vi "Example_IV_Curves.vi"() -> ()   [LabVIEW 2016]
uses:
  LockinDAQ/Typedefs/AO-cluster.ctl
  LockinDAQ/Typedefs/Function-enum.ctl
  Instrument.Lockin/Instrument.Lockin.lvclass
  <userlib>/LevyLab/LV to ITX/LVtoITX.lvclass
  LockinDAQ/Typedefs/AO_Channel-Numeric.ctl
  LockinDAQ/LockinDAQ.lvclass
panel:
  out "2 terminal":cluster{"Y":dbl[], "Y":dbl[]}(graph)
  out "4 terminal":cluster{"Y":dbl[], "Y":dbl[]}(graph)
  in  "step":dbl=0.025
  in  "end":dbl=0.1
  in  "start":dbl
  in  "Channels: AO":T1 {"f (Hz)" min=0.001 max=10000.0 format="%.3g"; "Phase (°)" format="%.3g"; "DC (V)" format="%.3p"; "Amp (V)" min=0.0 max=10.0 format="%.3p"}
  # "Lockin Example: IV Curves\nMake Sure Lockin Program is running!"
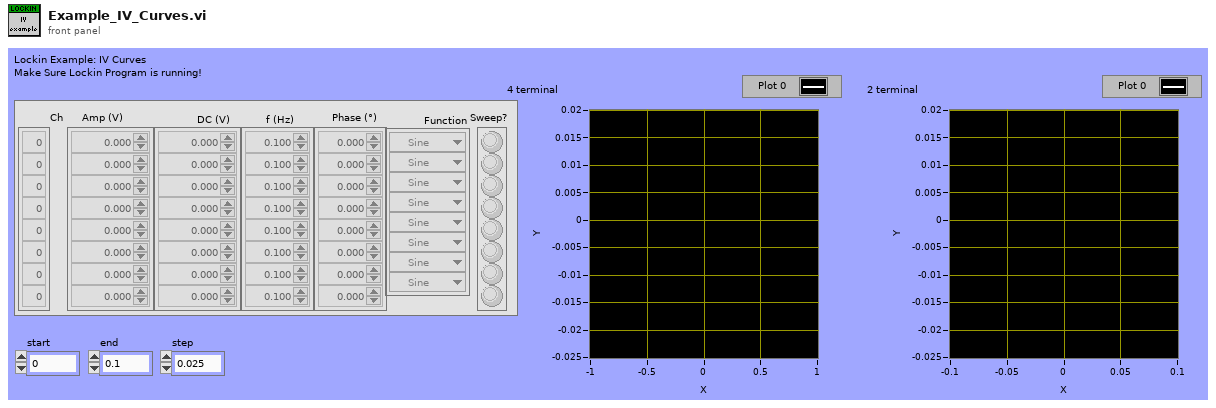
[diagram p1: front panel]
types:
  T1 = typedef "LockinDAQ.lvclass/AO-cluster.ctl" = cluster{"Ch":i32[], "Amp (V)":dbl[], "DC (V)":dbl[], "f (Hz)":dbl[], "Phase (°)":dbl[], "Function":T2[], "Sweep?":bool[]}
  T2 = typedef "LockinDAQ.lvclass/Function-enum.ctl" = enum16{"Sine", "Triangle", "Square", "Sawtooth"}
  T3 = typedef "LockinDAQ.lvclass/AO_Channel-Numeric.ctl" = i32
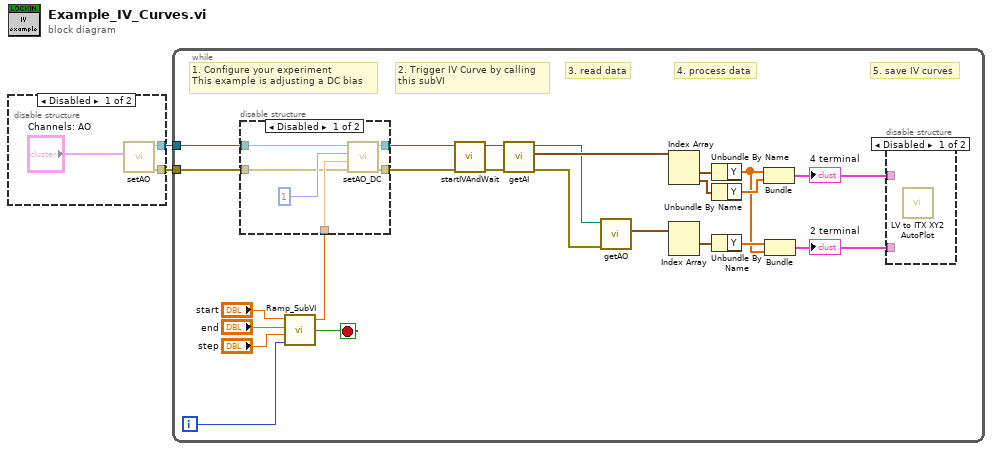
[diagram p0: block diagram]
diagram:
  n1 = disable-structure shown="Disabled" {
    disable-tunnel: [w4 _] -> w2
    disable-tunnel: [w3 _] -> w1
    frame Disabled {
      n2 = call "setAO.vi"("Channels: AO"="Channels: AO") -> ("error out"=w3:errorcluster, "Instrument.Lockin out"=w4:refnum<class "Instrument.Lockin.lvclass">)  [unwired: 9 in]
    }
    frame Enabled {
    }
  }
  n3 = while {
    tunnel: w2 -> [w14]
    tunnel: w1 -> [w13]
    i -> [w26]
    stop <- w29 stop-if-true
    # "5. save IV curves"
    # "4. process data"
    # "3. read data"
    # "1. Configure your experiment\nThis example is adjusting a DC bias"
    # "2. Trigger IV Curve by calling\nthis subVI"
    n4 = call <userlib>:"Ramp_SubVI.vi"("index"=w26, "step"="step", "end"="end", "start"="start") -> ("Stop?"=w29:bool, "Numeric"=w17:dbl)  [unwired: 1 in]
    n5 = disable-structure shown="Disabled" {
      disable-tunnel: w17 -> [w35 _]
      disable-tunnel: w14 -> [w33 _]
      disable-tunnel: w13 -> [w32 _]
      disable-tunnel: [w31 _] -> w12
      disable-tunnel: [w30 _] -> w11
      frame Disabled {
        n6 = call "setAO_DC.vi"("error in (no error)"=w32, "DC (V)"=w35, "AO Channel"=T3 1, "Instrument.Lockin in"=w33) -> ("error out"=w31:errorcluster, "Instrument.Lockin out"=w30:refnum<class "Instrument.Lockin.lvclass">)  [unwired: 6 in]
      }
      frame Enabled {
      }
    }
    n7 = call "startIVAndWait.vi"("error in (no error)"=w12, "Instrument.Lockin in"=w11) -> ("error out"=w9:errorcluster, "Instrument.Lockin out"=w10:refnum<class "Instrument.Lockin.lvclass">)  [unwired: 7 in, 1 out]
    n8 = call "getAI.vi"("error in (no error)"=w9, "Instrument.Lockin in"=w10) -> ("error out"=w8:errorcluster, "AI Waveform"=w15:waveform(dbl)[], "Instrument.Lockin out"=w7:refnum<class "Instrument.Lockin.lvclass">)  [unwired: 7 in]
    n9 = call "getAO.vi"("error in (no error)"=w8, "Instrument.Lockin in"=w7) -> ("AO Waveforrm"=w16:waveform(dbl)[])  [unwired: 7 in, 2 out]
    n10 = Index Array(array=w15) -> (element #1=w24:waveform(dbl), element #2=w23:waveform(dbl))  [unwired: 2 in]
    n11 = Index Array(array=w16) -> (element #1=w22:waveform(dbl))  [unwired: 2 in, 1 out]
    n12 = Unbundle By Name(w24) -> ("Y"=w6:dbl[])
    n13 = Unbundle By Name(w23) -> ("Y"=w21:dbl[])
    n14 = Unbundle By Name(w22) -> ("Y"=w20:dbl[])
    n15 = Bundle("Y"=w6, "Y"=w21) -> (w19:cluster{"Y":dbl[], "Y":dbl[]})  [unwired: 1 in]
    "4 terminal" <- w19
    n16 = Bundle("Y"=w20, "Y"=w6) -> (w18:cluster{"Y":dbl[], "Y":dbl[]})  [unwired: 1 in]
    "2 terminal" <- w18
    n17 = disable-structure shown="Disabled" {
      disable-tunnel: w19 -> [_ _]
      disable-tunnel: w18 -> [_ _]
      frame Disabled {
        n18 = call <userlib>:"LV to ITX XY2 AutoPlot.vi"() -> ()  [unwired: 15 in, 1 out]
      }
      frame Enabled {
      }
    }
  }
